vi "Fit_2D_GL.vi"(2 "Action":u16(ring) items=["Read Fit Data", "Fit Image"], 7 "Image IN":sgl[][](array[numeric])) -> (4 "Lorentz Fit Parameters":dbl[](array[numeric]), 6 "Lorentzian Image":dbl[][](array[numeric]), 8 "Gaussian Fit Parameters":dbl[](array[numeric]), 10 "Gaussian Image":dbl[][](array[numeric]), 13 "FitError":errorcluster)   [LabVIEW 2014]
uses:
  <vilib>/gmath/NumericalOptimization/Nonlinear Curve Fit LM.vi
  <vilib>/gmath/NI_Gmath.lvlib
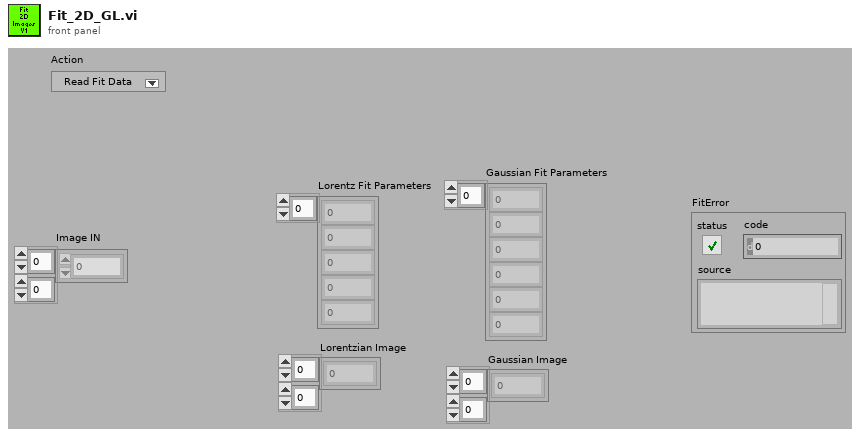
[diagram p1: front panel]
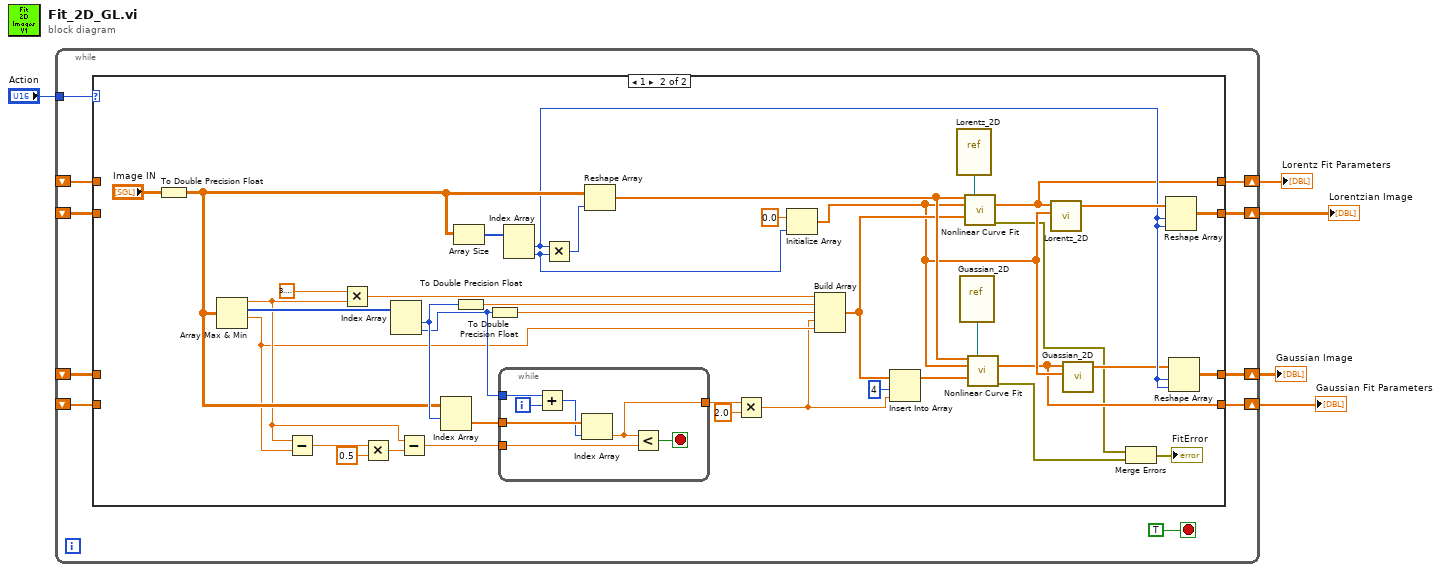
[diagram p0: block diagram]
diagram:
  n1 = while {
    tunnel: "Action" -> [w15]
    shift-right: [w10] -> w1
    shift-left: _ -> [w9]
    shift-right: [w13] -> w2
    shift-left: _ -> [w8]
    shift-right: [w12] -> w3
    shift-left: _ -> [w7]
    shift-right: [w11] -> w4
    shift-left: _ -> [w6]
    stop <- TRUE stop-if-true
    n2 = case shown="1" w15 {
      tunnel: [w18 w27] -> w13
      tunnel: [w17 w26] -> w12
      tunnel: [w16 w24] -> w11
      tunnel: [w19 w23] -> w10
      tunnel: w9 -> [w19 _]
      tunnel: w8 -> [w18 _]
      tunnel: w7 -> [w17 _]
      tunnel: w6 -> [w16 _]
      frame 0, Default {
      }
      frame 1 {
        n3 = To Double Precision Float(number="Image IN") -> (double precision float=w41:dbl[][])
        n4 = Array Max & Min(array=w41) -> (max value=w40:dbl, max index (indices)=w54:i32[], min value=w39:dbl)  [unwired: 1 out]
        n5 = Subtract(x=w40, y=w39) -> (x-y=w45:dbl)
        n6 = Multiply(x=3.141592653589793, y=w40) -> (x*y=w55:dbl)
        n7 = Multiply(x=w45, y=0.5) -> (x*y=w44:dbl)
        n8 = Index Array(array=w54) -> (element #1=w51:i32, element #2=w50:i32)  [unwired: 2 in]
        n9 = Subtract(x=w40, y=w44) -> (x-y=w48:dbl)
        n10 = Index Array(array=w41, index (row)=w51) -> (element=w49:dbl[])  [unwired: 1 in]
        n11 = Array Size(array=w41) -> (size(s)=w58:i32[])
        n12 = To Double Precision Float(number=w51) -> (double precision float=w53:dbl)
        n13 = To Double Precision Float(number=w50) -> (double precision float=w52:dbl)
        n14 = while {
          tunnel: w50 -> [w65]
          tunnel: w49 -> [w66]
          tunnel: w48 -> [w62]
          tunnel: [w60] -> w47
          i -> [w64]
          stop <- w61 stop-if-true
          n15 = Add(x=w65, y=w64) -> (x+y=w63:i32)
          n16 = Index Array(array=w66, index=w63) -> (element=w60:dbl)
          n17 = Less?(x=w60, y=w62) -> (x < y?=w61:bool)
        }
        n18 = Index Array(array=w58) -> (element #1=w28:i32, element #2=w37:i32)  [unwired: 2 in]
        n19 = Multiply(x=w28, y=w37) -> (x*y=w57:i32)
        n20 = Reshape Array(w41, w57) -> (w32:dbl[])
        n21 = Multiply(x=w47, y=2.0) -> (x*y=w35:dbl)
        n22 = Initialize Array(0.0 ("element"), w37) -> (w29:dbl[])
        n23 = Build Array(w55, w53, w52, w35, w39) -> (w31:dbl[])
        n24 = Insert Into Array(array=w31, index=4, new element=w35) -> (w33:dbl[])
        n25 = vi-ref "Lorentz_2D.vi"() -> (w42:refnum<vi>)
        n26 = vi-ref "Guassian_2D.vi"() -> (w34:refnum<vi>)
        n27 = call-poly <vilib>:"Nonlinear Curve Fit.vi"("Y"=w32, "f(x,a)"=w42, "X"=w29, "initial parameters"=w31) -> ("best fit parameters"=w23:dbl[], "error out"=w21:errorcluster)  [unwired: 6 in, 4 out]
        n28 = call-poly <vilib>:"Nonlinear Curve Fit.vi"("Y"=w32, "f(x,a)"=w34, "X"=w29, "initial parameters"=w33) -> ("best fit parameters"=w24:dbl[], "error out"=w22:errorcluster)  [unwired: 6 in, 4 out]
        n29 = call "Lorentz_2D.vi"("X"=w29, "a"=w23) -> ("f(X,a)"=w30:dbl[])  [unwired: 2 in, 2 out]
        n30 = call "Guassian_2D.vi"("X"=w29, "a"=w24) -> ("f(X,a)"=w25:dbl[])  [unwired: 2 in, 2 out]
        n31 = Merge Errors(w21, w22) -> (→"FitError":errorcluster)
        n32 = Reshape Array(w30, w28, w28) -> (w27:dbl[][])
        n33 = Reshape Array(w25, w28, w28) -> (w26:dbl[][])
      }
    }
  }
  "Lorentzian Image" <- w2
  "Gaussian Image" <- w3
  "Lorentz Fit Parameters" <- w1
  "Gaussian Fit Parameters" <- w4
